vi "ksENA Cap Meas Demo.vi"() -> ()   [LabVIEW 2013]
uses:
  Controls/Meas Type.ctl
panel:
  in  "Meas Type":T1
  in  "stop":bool
  out "P3":dbl[](graph)
  out "CPD":dbl[](graph)
  out "P2":dbl[](graph)
  out "P1":dbl[](graph)
  in  "VISA resource name":refnum<visa-resource-name>="E5080A"
  in  "Averaging Count":i32=3
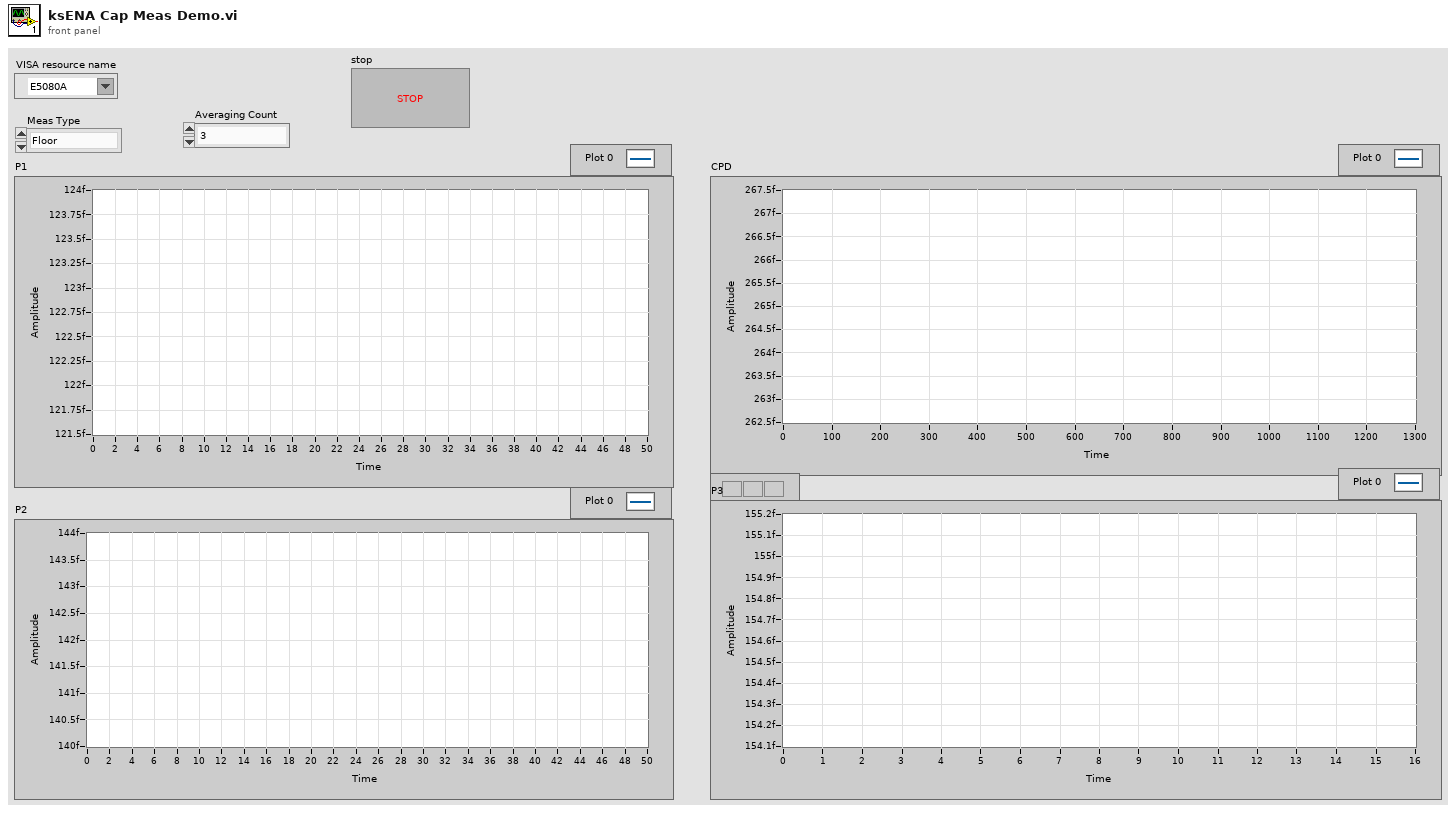
[diagram p1: front panel]
types:
  T1 = typedef "Meas Type.ctl" = enum16{"Floor", "Roof", "Buckling", "Charge Transfer"}
  T2 = typedef "ENA_Marker Measurements.ctl" = cluster{"Port 1 Capacitance":dbl[], "Port 2 Capacitance":dbl[], "Port 3 Capacitance":dbl[], "Port 1_S_parm":string[], "Port 2_S_parm":string[], "Port 3_S_parm":string[]}
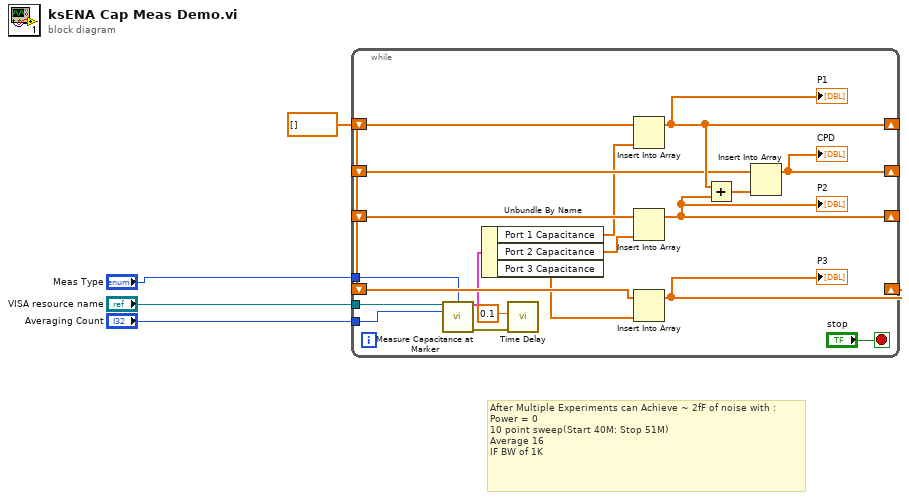
[diagram p0: block diagram]
diagram:
  w2 = dbl[] []
  # "After Multiple Experiments can Achieve ~ 2fF of noise with :\nPower = 0\n10 point sweep(Start 40M: Stop 51M)\nAverage 16\nIF BW of 1K"
  n1 = while {
    tunnel: "Averaging Count" -> [w23]
    tunnel: "VISA resource name" -> [w22]
    shift-right: [w19] -> _
    shift-left: w2 -> [w21]
    shift-right: [w15] -> _
    shift-left: w2 -> [w20]
    shift-right: [w14] -> _
    shift-left: w2 -> [w17]
    shift-right: [w13] -> _
    shift-left: w2 -> [w16]
    tunnel: "Meas Type" -> [w11]
    stop <- "stop" stop-if-true
    n2 = call "Measure Capacitance at Marker.vi"("VISA resource name"=w22, "Meas Type"=w11, "Averaging Count"=w23) -> ("Marker Measurements"=w10:T2, "Error Out"=w6:errorcluster)  [unwired: 11 in]
    n3 = Unbundle By Name(w10) -> ("Port 1 Capacitance"=w9:dbl[], "Port 2 Capacitance"=w8:dbl[], "Port 3 Capacitance"=w7:dbl[])
    n4 = call "Time Delay"("error in (no error)"=w6, "Delay Time (s)"=0.1) -> ()  [unwired: 9 in, 1 out]
    n5 = Insert Into Array(array=w21, new element=w9) -> (w19:dbl[])  [unwired: 1 in]
    "P1" <- w19
    n6 = Insert Into Array(array=w20, new element=w8) -> (w15:dbl[])  [unwired: 1 in]
    "P2" <- w15
    n7 = Insert Into Array(array=w16, new element=w7) -> (w13:dbl[])  [unwired: 1 in]
    "P3" <- w13
    n8 = Add(x=w19, y=w15) -> (x+y=w18:dbl[])
    n9 = Insert Into Array(array=w17, new element=w18) -> (w14:dbl[])  [unwired: 1 in]
    "CPD" <- w14
  }
